vi "StartUpGazebo.vi"() -> ()   [LabVIEW 2012]
panel:
  in  "telnet":string="192.168.1.13"
  out "Reply":string="--------------------------------------------------------------------------------\nNode [/turtlebot_node]\nPublications: \n * /imu/raw [sensor_msgs/Imu]\n * /rosout [rosgraph_msgs/Log]\n * /imu/data [sensor_msgs/Imu]\n * /diagnostics [diagnostic_msgs/DiagnosticArray]\n\nSubscriptions: None\n\nServices: None\n\n\ncontacting node http://130.64.94.183:39863/ ...\nPid: 22042\nConnections:\n * topic: /diagnostics\n    * to: /diagnostic_aggregator\n    * direction: outbound\n    * transport: TCPROS\n * topic: /rosout\n    * to: /rosout\n    * direction: outbound\n    * transport: TCPROS\n"
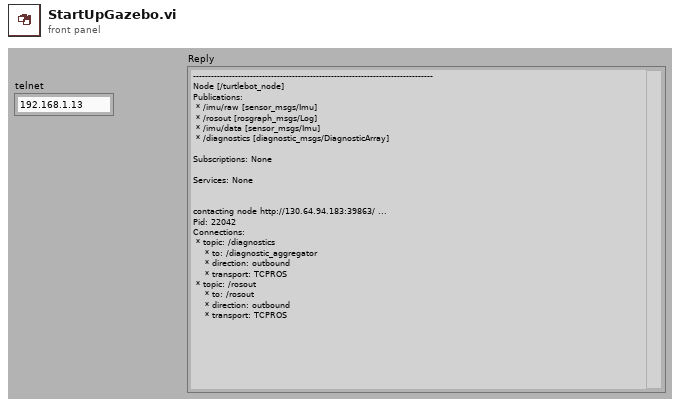
[diagram p1: front panel]
types:
  T1 = cluster{"Command":string, "Expected Reply":string}
  T2 = cluster{"Command":string, "Expected Reply":string}[]
  T3 = cluster{"IP":string, "Port":u16, "connection ID":refnum<k5>, "Host ERROR":bool, "timeout ms":i32, "buffer":string, "unfiltered buffer":string, "error":errorcluster}
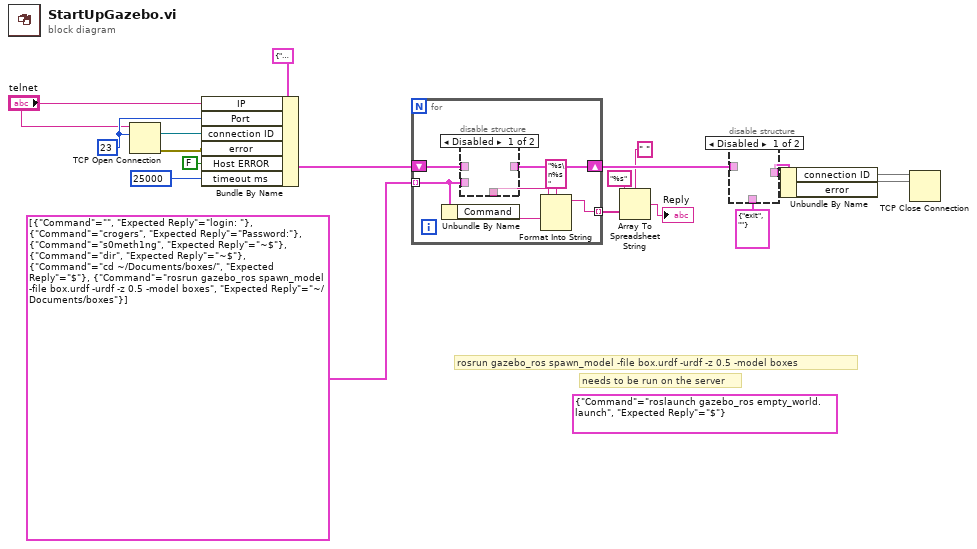
[diagram p0: block diagram]
diagram:
  (unwired) T1 {"Command"="roslaunch gazebo_ros empty_world.launch", "Expected Reply"="$"} ("Input")
  w15 = u16 23 ("remote port (23)")
  # "rosrun gazebo_ros spawn_model -file box.urdf -urdf -z 0.5 -model boxes"
  # "needs to be run on the server"
  n1 = TCP Open Connection(address="telnet", remote port or service name=w15) -> (connection ID=w17:refnum<k5>, error out=w16:errorcluster)  [unwired: 3 in]
  n2 = Bundle By Name(cluster=T3 {"IP"="", "Port"=0, "connection ID"=refnum, "Host ERROR"=FALSE, "timeout ms"=0, "buffer"="", "unfiltered buffer"="", "error"={"status"=FALSE, "code"=0, "source"=""}} ("ssh in"), "IP"="telnet", "Port"=w15, "connection ID"=w17, "error"=w16, "Host ERROR"=FALSE, "timeout ms"=u16 25000 ("remote port (23)")) -> (w10:T3)
  n3 = for {
    tunnel: [w21] -> w7 mode=indexing
    tunnel: T2 [{"Command"="", "Expected Reply"="login: "}, {"Command"="crogers", "Expected Reply"="Password:"}, {"Command"="s0meth1ng", "Expected Reply"="~$"}, {"Command"="dir", "Expected Reply"="~$"}, {"Command"="cd ~/Documents/boxes/", "Expected Reply"="$"}, {"Command"="rosrun gazebo_ros spawn_model -file box.urdf -urdf -z 0.5 -model boxes", "Expected Reply"="~/Documents/boxes"}] -> [w20] mode=indexing
    shift-right: [w25] -> w11
    shift-left: w10 -> [w24]
    n4 = Unbundle By Name(w20) -> ("Command"=w19:string)
    n5 = disable-structure shown="Disabled" {
      disable-tunnel: [_ _] -> w25
      disable-tunnel: w24 -> [_ _]
      disable-tunnel: [_ _] -> w22
      disable-tunnel: w20 -> [_ _]
      frame Disabled {
      }
      frame Enabled {
      }
    }
    n6 = Format Into String(format string="%s\n%s", w19, w22) -> (resulting string=w21:string)  [unwired: 2 in, 1 out]
  }
  n7 = Array To Spreadsheet String(delimiter (Tab)=" ", array=w7, 3:"%s" ("format string")) -> (spreadsheet string=→"Reply":string)
  n8 = disable-structure shown="Disabled" {
    disable-tunnel: w11 -> [_ _]
    disable-tunnel: T1 {"Command"="exit", "Expected Reply"=""} ("Input") -> [_ _]
    disable-tunnel: [_ _] -> w3
    frame Disabled {
    }
    frame Enabled {
    }
  }
  n9 = Unbundle By Name(w3) -> ("connection ID"=w2, "error"=w1)
  n10 = TCP Close Connection(connection ID=w2, error in (no error)=w1) -> ()  [unwired: 3 out]
